vi "小三轮的 FPGA Main Default.vi"() -> ()   [LabVIEW 2017]
doc: "The myRIO v1.1 FPGA Shipping Personality. This personality contains support for:\n- 2 Analog Input Interrupt channel\n- 4 Digital Input Interrupt channel\n- 1 Timer\n- 1 Accelerometer\n- 1 Button\n- 4 LED\n- 10 Analog Input channels with 1 Sample\n- 6 Analog Output channels with 1 Sample\n- 40 Digital I/O channels with 1 Sample\n- 2 I2C channels\n- 4 Encoder channels\n- 6 PWM channels\n- 2 SPI channels"
uses:
  <vilib>/Platform/TimedLoop/XDataNode/timing_clust.ctl
  <vilib>/Platform/TimedLoop/XDataNode/nitl_modes.ctl
  <vilib>/Platform/TimedLoop/XDataNode/wakeup.ctl
  <vilib>/rvi/Emulation/niFpgaGetClockAttributes.vi
  <vilib>/rvi/Emulation/niFpgaSctlEmulationGetInTimedLoop.vi
  <vilib>/rvi/Emulation/niFpgaEmulationReportErrorSimple.vi
  <vilib>/rvi/eio/common/nirviEmuTemplateMethod_errors.vi
  <vilib>/rvi/Emulation/niFpgaCriticalErrorInLSC.vi
  <vilib>/rvi/Emulation/niFpgaProcessEmulError.vi
  <vilib>/rvi/Emulation/niFpgaEmulationIsFPGAContextNoSignature.vi
  <vilib>/rvi/errors/niFpgaSetErrorForExecOnDevCompSimple.vi
  <vilib>/rvi/eio/common/nirviEmuReportErrorAndStop.vi
  <vilib>/rvi/DataTransferAndStorage/Container/Common/niFpgaContainerGetUniqueNameForEmu.vi
  <vilib>/rvi/FIFO/Fifo_Resource/nirvififoEmulationSetSize.vi
  <vilib>/rvi/FIFO/Fifo_Resource/nirviFifoEmulationQueueMgr.vi
  <instcachedir>/0/nirviFifoEmulationQueueMgr_E5CAEC123FF24DC58D834DCA3CDAA9B5.lvgen/nirviFifoEmulationQueueMgr_E5CAEC123FF24DC58D834DCA3CDAA9B5_002.vi
  <vilib>/rvi/FIFO/Fifo_Resource/nirvififoEmulationDetermineInputValidOut.vi
  <vilib>/rvi/FIFO/Fifo_Resource/nirvififoEmulationCreateLock.vi
  <vilib>/rvi/FIFO/Fifo_Resource/nirvififoEmulationObtainLock.vi
  <vilib>/rvi/FIFO/Fifo_Resource/nirvififoEmulationReleaseLock.vi
  <vilib>/rvi/occurrence/nirviWaitOnOccurrenceBase.vi
  <vilib>/rvi/errors/nirviReportUnexpectedCaseInternalError.vi
  <vilib>/rvi/errors/nirviReportUnexpectedCaseInternalError (U32).vi
  <vilib>/Utility/error.llb/Clear Errors.vi
  <vilib>/rvi/DataTransferAndStorage/Container/Common/niFpgaContainerSetEmuInfo.vi
  <vilib>/eio/EIONode/EIONode.xnode
  <vilib>/rvi/DataTransferAndStorage/Container/XNode/niFpgaContainer.xnode
  <vilib>/rvi/FIFO/Fifo_Resource/nirvififoEmulationWrite.vi
  <vilib>/rvi/FIFO/Fifo_Resource/nirvififoEmulationRead.vi
  <vilib>/Platform/TimedLoop/XDataNode/XDataNode.xnode
  <vilib>/rvi/LocalResourceManager/LocalResourceManager.xnode
  <vilib>/Platform/TimedLoop/XDataNode/XDNodeRunTimeDep.lvlib
panel:
  out "timed out? 2":bool
  out "pulse width (uSec) 2":u32
  out "pulse width (uSec)":u32
  out "timed out?":bool
  in  "Reset ENC":bool
  out "ENC2":i32
  out "ENC1":i32
  in  "AO.A_0.VAL":u16
  in  "AO.A_1.VAL":u16
  in  "AO.B_0.VAL":u16
  in  "AO.B_1.VAL":u16
  out "AI.B_3.VAL":u16
  out "AI.B_2.VAL":u16
  out "AI.B_1.VAL":u16
  out "AI.B_0.VAL":u16
  out "AI.A_3.VAL":u16
  out "AI.A_2.VAL":u16
  out "AI.A_1.VAL":u16
  out "AI.A_0.VAL":u16
  out "DIO.B_7:0.IN":u8 format="%08b"
  in  "DIO.B_7:0.DIR":u8 format="%08b"
  in  "DIO.B_7:0.OUT":u8 format="%08b"
  in  "PWM.A_2.CS":u8=1
  in  "PWM.A_2.CNFG":u8=4
  out "PWM.A_2.CNTR":u16
  in  "PWM.A_2.MAX":u16=39999
  in  "PWM.A_2.CMP":u16=20000
  in  "PWM.A_1.CS":u8=1
  in  "PWM.A_1.CNFG":u8=4
  out "PWM.A_1.CNTR":u16
  in  "PWM.A_1.MAX":u16=39999
  in  "PWM.A_1.CMP":u16=20000
  in  "PWM.A_0.CS":u8=1
  in  "PWM.A_0.CNFG":u8=4
  out "PWM.A_0.CNTR":u16
  in  "PWM.A_0.CMP":u16=20000
  in  "PWM.A_0.MAX":u16=39999
  in  "SPI.A.DATO":u16
  out "SPI.A.DATI":u16
  in  "SPI.A.CNFG":u16=112
  in  "SPI.A.CNT":u16=19
  in  "SPI.B.CNT":u16=19
  in  "SPI.B.CNFG":u16=112 format="%0.0f"
  out "SPI.B.DATI":u16
  in  "SPI.B.DATO":u16
  in  "ENC.A.CNFG":u8 format="%08b"
  in  "ENC.B.CNFG":u8 format="%08b"
  out "ENC.A.CNTR":u32
  out "ENC.B.CNTR":u32
  out "ENC.A.STAT":u8 format="%08b"
  out "ENC.B.STAT":u8 format="%08b"
  in  "SPI.A.GO":T1
  out "SPI.A.STAT":u8 format="%08b"
  in  "SPI.B.GO":T1
  out "SPI.B.STAT":u8 format="%08b"
  out "I2C.B.STAT":u8 format="%08b"
  in  "I2C.B.CNTL":u8 format="%08b"
  out "I2C.A.STAT":u8 format="%08b"
  in  "I2C.A.CNTL":u8 format="%08b"
  in  "I2C.B.CNTR":u8=213
  in  "I2C.B.ADDR":u8 format="%08.0f"
  out "I2C.B.DATI":u8
  in  "I2C.B.DATO":u8
  in  "I2C.A.CNTR":u8=213
  in  "I2C.A.ADDR":u8 format="%08b"
  out "I2C.A.DATI":u8
  in  "I2C.A.DATO":u8
  in  "I2C.B.CNFG":u8=1 format="%08b"
  in  "I2C.A.CNFG":u8=1 format="%08b"
  in  "I2C.A.GO":T1
  in  "I2C.B.GO":T1
  out "SYS.AI.RDY":bool
  out "SYS.RDY":bool
  in  "PWM.B_2.CS":u8=1
  in  "PWM.B_2.CNFG":u8=4
  out "PWM.B_2.CNTR":u16
  in  "PWM.B_2.MAX":u16=39999
  in  "PWM.B_2.CMP":u16=20000
  in  "PWM.B_1.CS":u8=1
  in  "PWM.B_1.CNFG":u8=4
  out "PWM.B_1.CNTR":u16
  in  "PWM.B_1.MAX":u16=39999
  in  "PWM.B_1.CMP":u16=20000
  in  "PWM.B_0.CS":u8=1
  in  "PWM.B_0.CNFG":u8=4
  out "PWM.B_0.CNTR":u16
  in  "PWM.B_0.MAX":u16=39999
  in  "PWM.B_0.CMP":u16=20000
  out "DIO.A_7:0.IN":u8 format="%08b"
  in  "DIO.A_7:0.OUT":u8 format="%08b"
  in  "DIO.A_7:0.DIR":u8 format="%08b"
  out "DIO.C_7:0.IN":u8 format="%08b"
  in  "DIO.C_7:0.DIR":u8 format="%08b"
  in  "DIO.C_7:0.OUT":u8 format="%08b"
  out "AI.C_1.VAL":u16
  out "AI.C_0.VAL":u16
  in  "AO.C_0.VAL":u16
  in  "AO.C_1.VAL":u16
  in  "SYS.SELECTB":u8 format="%08b"
  in  "SYS.SELECTC":u8 format="%08b"
  in  "SYS.SELECTA":u8 format="%08b"
  in  "ENC.C_0.CNFG":u8 format="%08b"
  out "ENC.C_0.CNTR":u32
  out "ENC.C_0.STAT":u8 format="%08b"
  in  "ENC.C_1.CNFG":u8 format="%08b"
  out "ENC.C_1.CNTR":u32
  out "ENC.C_1.STAT":u8 format="%08b"
  in  "PWM.C_1.CS":u8=1
  in  "PWM.C_1.CNFG":u8=4
  out "PWM.C_1.CNTR":u16
  in  "PWM.C_1.CMP":u16=20000
  in  "PWM.C_1.MAX":u16=39999
  in  "PWM.C_0.CS":u8=1
  in  "PWM.C_0.CNFG":u8=4
  out "PWM.C_0.CNTR":u16
  in  "PWM.C_0.CMP":u16=20000
  in  "PWM.C_0.MAX":u16=39999
  out "DIO.A_15:8.IN":u8 format="%08b"
  in  "DIO.A_15:8.OUT":u8 format="%08b"
  in  "DIO.A_15:8.DIR":u8 format="%08b"
  out "DIO.B_15:8.IN":u8 format="%08b"
  in  "DIO.B_15:8.DIR":u8 format="%08b"
  in  "DIO.B_15:8.OUT":u8 format="%08b"
  out "AI.AudioIn_R.VAL":u16
  out "AI.AudioIn_L.VAL":u16
  in  "AO.AudioOut_R.VAL":u16
  in  "AO.AudioOut_L.VAL":u16
  in  "AO.SYS.GO":T1
  out "AO.SYS.STAT":bool
  in  "IRQ.AI_A_3:0.CNFG":u8 format="%.0b"
  in  "IRQ.AI_A_0.THRESHOLD":u16
  in  "IRQ.AI_A_1.THRESHOLD":u16
  in  "IRQ.AI_A_0.NO":u8
  in  "IRQ.AI_A_1.NO":u8
  in  "IRQ.DIO_A_7:0.ENA":u8 format="%08b"
  in  "IRQ.DIO_A_7:0.RISE":u8 format="%08b"
  in  "IRQ.DIO_A_7:0.FALL":u8 format="%08b"
  in  "IRQ.DIO_A_0.NO":u8
  in  "IRQ.DIO_A_1.NO":u8
  in  "IRQ.DIO_A_2.NO":u8
  in  "IRQ.DIO_A_3.NO":u8
  in  "IRQ.DIO_A_3.CNT":u32
  in  "IRQ.DIO_A_2.CNT":u32
  in  "IRQ.DIO_A_1.CNT":u32
  in  "IRQ.DIO_A_0.CNT":u32
  in  "IRQ.AI_A_1.HYSTERESIS":u16=17
  in  "IRQ.TIMER.WRITE":u32
  in  "IRQ.TIMER.SETTIME":T1
  out "IRQ.TIMER.READ":u32
  in  "SPI.A.IRQ.NO":u8=15
  in  "SPI.B.IRQ.NO":u8=15
  in  "IRQ.AI_A_0.HYSTERESIS":u16=17
  # "System"
  # "Onboard Devices"
  # "Connector A"
  # "Connector B"
  # "Connector C"
  # "Audio Connector"
  # "Accelerometer"
  # "Analog Input"
  # "Analog Output"
  # "Digital I/O"
  # "PWM"
  # "SPI Master"
  # "Analog Input"
  # "Analog Output"
  # "Digital I/O"
  # "PWM"
  # "SPI Master"
  # "Analog Input"
  # "Analog Output"
  # "Digital I/O"
  # "Counters / PWM"
  # "Analog Input"
  # "Analog Output"
  # "IO Configuration"
  # "IO Configuration"
  # "IO Configuration"
  # "Encoders"
  # "Buttons & LEDs"
  # "Analog Interrupt"
  # "Digital Interrupt"
  # "Encoders"
  # "Encoders"
  # "Button Interrupt"
  # "I2C Master"
  # "I2C Master"
  # "Timer Interrupt"
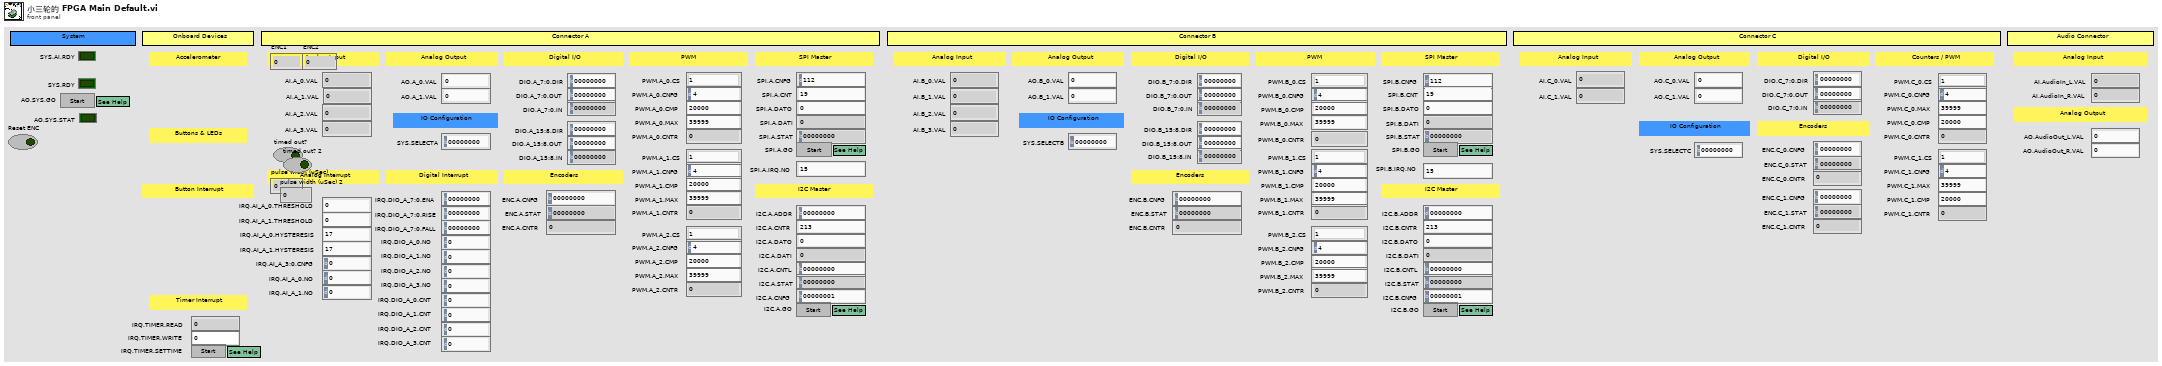
[diagram p1: front panel]
types:
  T1 = typedef "小三轮的 Start Boolean.ctl" = bool
  T2 = typedef "XDNodeRunTimeDep.lvlib/timing_clust.ctl" = cluster{"Expected End [f-1]":u64, "Actual End [f-1]":u64, "Finished Late? [f-1]":bool, "Expected End [i-1]":u64, "Actual End [i-1]":u64, "Finished Late? [i-1]":bool, "Expected Start [i]":u64, "Actual Start [i]":u64, "Expected Start [f]":u64, "Actual Start [f]":u64, "Source Name":string, "Structure Name":string, "Period":i64, "Deadline":i64, "Offset":i64, "Start":i64, "Priority":i32, "Timeout":i32, "Mode":T3, "Wakeup Reason":T4, "Error":errorcluster, "Source Type":string, "Secondary Source Type":string, "Global End Time":u64, "Global Start Time":u64, "Frame Duration":u64, "Iteration Duration":u64, "Assigned CPU":i32, "I/O Scan Engine Mode":u32}
  T3 = typedef "XDNodeRunTimeDep.lvlib/nitl_modes.ctl" = enum32{"No Change", "Process missed periods, maintain original phase", "Discard missed periods, maintain original phase", "Process missed periods, ignore original phase", "Discard missed periods, ignore original phase"}
  T4 = typedef "XDNodeRunTimeDep.lvlib/wakeup.ctl" = enum32{"Normal", "Aborted", "Asynchronous wakeup", "Timing source error", "Timed loop error", "Timeout"}
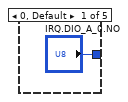
[diagram p6: hidden frame]
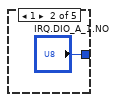
[diagram p7: hidden frame]
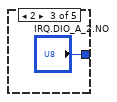
[diagram p8: hidden frame]
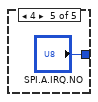
[diagram p9: hidden frame]
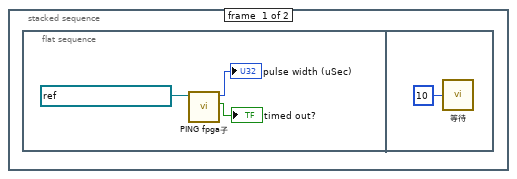
[diagram p10: hidden frame]
diagram:
  # "The Timed Loop does not allow writing the same FIFO outside the Timed Loop. Use another FIFO to push all interrupts from DIO in the Timed Loop to the IRQ Queue."
  # "The Timed Loop does not allow writing the same FIFO outside the Timed Loop. Use another FIFO to push all interrupts from DIO in the Timed Loop to the IRQ Queue."
  # "The analog output nodes take some time before the FPGA write the values to the pins. The GO and STAT registers are used to handshake between the FPGA and host. When the host wants the values to be written, the host sets the GO register to TRUE. If the host reads the STAT register before setting the value of the GO register, it can wait for the value of the STAT register to invert. The value inversion tells the host that the output values have been written."
  # "The analog input nodes take some time before the FPGA can first read the values. This is because it takes time to set up the Analog-to-Digital converter (ADC) and convert the first reading. An iteration of the While Loop will not complete until all the analog input channels have been sampled.\n\nAfter the completion of the first iteration of the While Loop, all indicators have valid values."
  # "Note: On some hardware a \"ghosting effect\" may occur on any unconnected AI channels. For example, if channel AI0 is connected and channels AI1~AI7 are not connected the the value read at AI0 may be seen on indicators AI1~AI7. This is common for hardware that use a multiplexed (MUXed) Analog-to-Digital converter (ADC), because the input analog signal is used to charge a capacitor which does not discharge before the unconnected channel is read.\n\nYou can hide the \"ghosting effect\" by using an mask register. This register is used to decide when the indicator should be updated."
  # "The FPGA timer fires the interrupt request (IRQ) when TIMER.Read counts down to zero. If TIMER.Read is not zero, it counts down to one per microsecond."
  # "The only interface that sends interrupts to the RT side. Timer interrupts, analog input interrupts, digital input interrupts, and SPI interrupt share this interface.\n\nAll interrupts work in sequence. One interrupt waits until the previous interrupt request (IRQ) gets acknowledged on the RT side."
  # "NOTE: The SYS.RDY Boolean MUST exist and must become TRUE at some point. Otherwise, the myRIO VIs will not function correctly."
  # "There is some delay between the time when the FPGA code starts and the time when the analog inputs, accelerometer, and scaling values outputs are valid. If the host wants to ensure that there are valid values in theses registers it should wait for each subsystem to finish its initialization process. \n\nWhen all subsystems have finished initializinig, the SYS.RDY indicator turns true. The host can poll the SYS.RDY indicator to determine the status of the FPGA. Alternatively, the host can poll the individual SYS.xx.RDY indicators to determine the status of the individual subsystems.\n\nThis loop continues indefinitely, essentially making SYS.RDY a read-only register."
  n1 = while {
    stop <- FALSE stop-if-true
    # "Host Synchronization"
    n2 = local read "SYS.AI.RDY"() -> (→"SYS.RDY":bool)
  }
  n3 = while {
    stop <- FALSE stop-if-true
    # "Interrupt to RT"
    n4 = xnode ("FIFO Method Node")("超时"=-1 ("Timeout")) -> ("元素"=w13:u8)  [unwired: 1 in, 2 out]
    n5 = call <vilib>:"niFPGA Interrupt.vi"("Wait Until Cleared (F)"=TRUE, "IRQ Number (0)"=w13) -> ()  [unwired: 1 in]
  }
  n6 = while {
    stop <- FALSE stop-if-true
    # "Timer"
    n7 = local read "IRQ.TIMER.READ"() -> (w18:u32)
    n8 = Select(t="IRQ.TIMER.WRITE", s="IRQ.TIMER.SETTIME", f=w18) -> (s? t:f=w16:u32)
    n9 = case shown="默认" w16 {
      selector: w16 -> [w22 w25]
      tunnel: [w22 w23] -> w15
      frame 0 {
      }
      frame Default {
        n10 = Decrement(x=w25) -> (x-1=w24:u32)
        n11 = case shown="0" w24 {
          selector: w24 -> [w26 w29]
          tunnel: [w26 w29] -> w23
          frame Default {
          }
          frame 0 {
            w28 = u8 0  # Reserved for Timer IRQ
            n12 = xnode ("FIFO Method Node")("元素"=w28, "超时"=-1 ("Timeout")) -> ()  [unwired: 1 in, 2 out]
          }
        }
      }
    }
    "IRQ.TIMER.READ" <- w15
    n13 = call "Loop Timer"("Count(uSec)"=u8 1 ("Count(mSec)")) -> ()  [unwired: 1 out]
  }
  n14 = xnode "通过VI定义FIFO配置"() -> ("FIFO输出"=w2:refnum<k21>)
  n15 = while {
    tunnel: w2 -> [w31]
    i -> [w58]
    stop <- FALSE stop-if-true
    # "Analog Input"
    n16 = xnode "FPGA I/O节点"() -> ("ConnectorA/AI0"=w36:u16, "ConnectorA/AI1"=w35:u16, "ConnectorA/AI2"=→"AI.A_2.VAL":u16, "ConnectorA/AI3"=→"AI.A_3.VAL":u16, "ConnectorB/AI0"=→"AI.B_0.VAL":u16, "ConnectorB/AI1"=→"AI.B_1.VAL":u16, "ConnectorB/AI2"=→"AI.B_2.VAL":u16, "ConnectorB/AI3"=→"AI.B_3.VAL":u16, "ConnectorC/AI0"=w52:i16, "ConnectorC/AI1"=w51:i16, "AudioIn/Left"=w50:i16, "AudioIn/Right"=w49:i16)  [unwired: 12 in, 12 out]
    "AI.A_0.VAL" <- w36
    "AI.A_1.VAL" <- w35
    n17 = Greater Than 0?(x=w58) -> (x > 0?=→"SYS.AI.RDY":bool)
    n18 = Number To Boolean Array(number="IRQ.AI_A_3:0.CNFG") -> (Boolean array=w46:bool[])
    n19 = Index Array(array=w46) -> (element #1=w44:bool, element #2=w43:bool, element #3=w41:bool, element #4=w40:bool)  [unwired: 4 in]
    n20 = To Unsigned Word Integer(number=w52) -> (unsigned 16bit integer=→"AI.C_0.VAL":u16)
    n21 = To Unsigned Word Integer(number=w51) -> (unsigned 16bit integer=→"AI.C_1.VAL":u16)
    n22 = To Unsigned Word Integer(number=w50) -> (unsigned 16bit integer=→"AI.AudioIn_L.VAL":u16)
    n23 = To Unsigned Word Integer(number=w49) -> (unsigned 16bit integer=→"AI.AudioIn_R.VAL":u16)
    n24 = call "小三轮的 Check AI IRQ.vi"("Hysteresis"="IRQ.AI_A_1.HYSTERESIS", "FIFO In"=w31, "IRQ Number"="IRQ.AI_A_1.NO", "Threshold"="IRQ.AI_A_1.THRESHOLD", "Analog Value"=w35, "Rising Edge?"=w40, "Enable Interrupt?"=w41) -> ()  [unwired: 5 in]
    n25 = call "小三轮的 Check AI IRQ.vi"("Hysteresis"="IRQ.AI_A_0.HYSTERESIS", "FIFO In"=w31, "IRQ Number"="IRQ.AI_A_0.NO", "Threshold"="IRQ.AI_A_0.THRESHOLD", "Analog Value"=w36, "Rising Edge?"=w43, "Enable Interrupt?"=w44) -> ()  [unwired: 5 in]
  }
  n26 = while {
    stop <- FALSE stop-if-true
    # "Analog Output"
    n27 = feedback #1(FALSE) -> (w64:bool)
    n28 = case shown="真" "AO.SYS.GO" {
      tunnel: "AO.C_0.VAL" -> [_ w86]
      tunnel: "AO.C_1.VAL" -> [_ w85]
      tunnel: "AO.A_0.VAL" -> [_ w90]
      tunnel: "AO.A_1.VAL" -> [_ w89]
      tunnel: "AO.B_0.VAL" -> [_ w88]
      tunnel: "AO.B_1.VAL" -> [_ w87]
      tunnel: "AO.AudioOut_L.VAL" -> [_ w82]
      tunnel: "AO.AudioOut_R.VAL" -> [_ w81]
      tunnel: w64 -> [w75 w78]
      tunnel: [w75 w76] -> w62
      frame False {
      }
      frame True {
        n29 = To Word Integer(number=w86) -> (16bit integer=w84:i16)
        n30 = To Word Integer(number=w85) -> (16bit integer=w83:i16)
        n31 = To Word Integer(number=w82) -> (16bit integer=w80:i16)
        n32 = To Word Integer(number=w81) -> (16bit integer=w79:i16)
        n33 = flat-sequence {
          tunnel: w90 -> [w99]
          tunnel: w89 -> [w98]
          tunnel: w88 -> [w97]
          tunnel: w87 -> [w96]
          tunnel: w84 -> [w95]
          tunnel: w83 -> [w94]
          tunnel: w80 -> [w93]
          tunnel: w79 -> [w92]
          tunnel: w78 -> [w91]
          tunnel: [w91] -> w77
          tunnel: w77 -> [w101]
          tunnel: [w100] -> w76
          frame #0 {
            n34 = xnode "FPGA I/O节点"("ConnectorA/AO0"=w99, "ConnectorA/AO1"=w98, "ConnectorB/AO0"=w97, "ConnectorB/AO1"=w96, "ConnectorC/AO0"=w95, "ConnectorC/AO1"=w94, "AudioOut/Left"=w93, "AudioOut/Right"=w92) -> ()  [unwired: 8 in, 8 out]
          }
          frame #1 {
            n35 = Not(x=w101) -> (.not. x?=w100:bool)
          }
        }
      }
    }
    "AO.SYS.STAT" <- w62
    n36 = feedback-in #1(w62) -> ()
  }
  n37 = while {
    stop <- FALSE stop-if-true
    # "PING)))"
    n38 = stacked-sequence {
      frame #0 {
        n39 = flat-sequence {
          frame #0 {
            n40 = call "PING fpga子.vi"("引用句柄输入"=refnum<k21> "ConnectorB/DIO0") -> ("timed out?"=→"timed out?":bool, "pulse width (uSec)"=→"pulse width (uSec)":u32)  [unwired: 9 in]
          }
          frame #1 {
            n41 = call "等待"("Count(uSec)"=u32 10) -> ()  [unwired: 1 out]
          }
        }
      }
      frame #1 {
        n42 = flat-sequence {
          frame #0 {
            n43 = call "PING fpga子.vi"("引用句柄输入"=refnum<k21> "ConnectorB/DIO1") -> ("timed out?"=→"timed out? 2":bool, "pulse width (uSec)"=→"pulse width (uSec) 2":u32)  [unwired: 9 in]
          }
          frame #1 {
            n44 = call "等待2"("Count(uSec)"=u32 10) -> ()  [unwired: 1 out]
          }
        }
      }
    }
  }
  n45 = while {
    stop <- FALSE stop-if-true
    # "Encode"
    n46 = xnode "FPGA I/O节点"() -> ("ConnectorA/DIO0"=w118:bool, "ConnectorA/DIO1"=w117:bool, "ConnectorA/DIO2"=w116:bool, "ConnectorA/DIO3"=w115:bool)  [unwired: 4 in, 4 out]
    n47 = call "FPGA Encode.vi"("Reset ENC1"="Reset ENC", "B"=w117, "A"=w118) -> ("ENC"=→"ENC1":i32)  [unwired: 8 in]
    n48 = call "FPGA Encode.vi"("Reset ENC1"="Reset ENC", "B"=w115, "A"=w116) -> ("ENC"=→"ENC2":i32)  [unwired: 8 in]
  }
  n49 = node-c288() -> (w6:T2)  [unwired: 1 in]
  n50 = xnode "通过VI定义FIFO配置"() -> ()  [unwired: 1 out]
  n51 = while {
    stop <- FALSE stop-if-true
    # "Connector A SCTL Interrupt Buffer"
    n52 = feedback #2(u8 0 ("Element")) -> (w121:u8)
    n53 = feedback #3(FALSE ("Timed Out?")) -> (w125:bool)
    n54 = case shown="假" w125 {
      tunnel: [w127 w129] -> w122
      tunnel: w121 -> [_ w129]
      frame False {
        n55 = xnode ("FIFO Method Node")("超时"=-1 ("Timeout")) -> ("元素"=w127:u8)  [unwired: 1 in, 2 out]
      }
      frame True {
      }
    }
    n56 = feedback-in #2(w122) -> ()
    n57 = xnode ("FIFO Method Node")("元素"=w122, "超时"=0 ("Timeout")) -> ("超时？"=w123:bool)  [unwired: 1 in, 1 out]
    n58 = feedback-in #3(w123) -> ()
  }
  n59 = timed-loop {
    timing: w6 -> [_]
    timing-out: [_] -> w5
    stop <- _ stop-if-true
    w153 = fxp<+,4,4> 0.0 ("IN 3:0")
    w130 = u16 5 ("Debounce Ticks")
    w131 = u8 0
    # "Trigger the interrupt at next \ntick if timeout"
    # "DIO / Encoder"
    # "DIO / I2C Master"
    # "DIO / PWM"
    # "DIO"
    # "DIO"
    # "DIO/ SPI Master"
    # "Connector A DIO"
    n60 = call "小三轮的 Split HDC Bank1 DIO.vi"("IN 7:0"="DIO.A_7:0.OUT") -> ("OUT 4"=w185:bool, "OUT 7:5"=w259:fxp<+,3,3>)  [unwired: 1 out]
    n61 = call "小三轮的 Split HDC Bank1 DIO.vi"("IN 7:0"="DIO.A_7:0.DIR") -> ("OUT 4"=w260:bool, "OUT 7:5"=w258:fxp<+,3,3>)  [unwired: 1 out]
    n62 = call "小三轮的 Split HDC Function Select.vi"("IN 7:0"="SYS.SELECTA") -> ("OUT 1:0"=w205:fxp<+,2,2>, "OUT 7"=w200:bool, "OUT 2"=w204:bool, "OUT 3"=w203:bool, "OUT 4"=w202:bool, "OUT 5"=w201:bool)
    n63 = call "小三轮的 DIO 1-bit.vi"("DIR"=w260, "OUT"=w185, "DIO Refnum"=refnum<k21> "ConnectorA/DIO4") -> ("IN"=w152:bool)  [unwired: 8 in]
    n64 = call "小三轮的 DIO_SPI.vi"("DIO.2:0.OUT"=w259, "DIO.2:0.DIR"=w258, "SPI.CNT"="SPI.A.CNT", "SPI.CNFG"="SPI.A.CNFG", "SPI.DATO"="SPI.A.DATO", "SPI.GO"="SPI.A.GO", "DIO.2/SPI.MOSI Refnum"=refnum<k21> "ConnectorA/DIO7" ("DIO.2/SPI.SCLK"), "SELECT.1:0"=w205, "DIO.1/SPI.MISO Refnum"=refnum<k21> "ConnectorA/DIO6" ("DIO.1/SPI.MOSI"), "DIO.0/SPI.SCLK Refnum"=refnum<k21> "ConnectorA/DIO5" ("DIO.0/SPI.MISO")) -> ("DIO.2:0.IN"=w238:fxp<+,3,3>, "SPI.DATI"=→"SPI.A.DATI":u16, "SPI.STAT"=w138:u8)  [unwired: 7 in]
    "SPI.A.STAT" <- w138
    n65 = Number To Boolean Array(number=w138) -> (Boolean array=w140:bool[])
    n66 = Index Array(array=w140) -> (element=w139:bool)  [unwired: 1 in]
    n67 = call "小三轮的 Falling Edge Trigger.vi"("Signal"=w139) -> ("Trigger?"=w137:bool)
    n68 = call "小三轮的 Join HDC Bank1 DIO.vi"("IN 7:5"=w238, "IN 4"=w152, "IN 3:0"=w153) -> ("OUT 7:0"=→"DIO.A_7:0.IN":u8)
    n69 = Number To Boolean Array(number=w153) -> (Boolean array=w178:bool[])
    n70 = Number To Boolean Array(number="IRQ.DIO_A_7:0.ENA") -> (Boolean array=w184:bool[])
    n71 = Number To Boolean Array(number="IRQ.DIO_A_7:0.RISE") -> (Boolean array=w183:bool[])
    n72 = Number To Boolean Array(number="IRQ.DIO_A_7:0.FALL") -> (Boolean array=w182:bool[])
    n73 = call "小三轮的 Split HDC Bank2 DIO.vi"("IN 7:0"="DIO.A_15:8.OUT") -> ("OUT 5"=w187:bool, "OUT 7:6"=w209:fxp<+,2,2>, "OUT 4:3"=w189:fxp<+,2,2>, "OUT 2"=w191:bool, "OUT 0"=w195:bool, "OUT 1"=w194:bool)  [unwired: 2 in]
    n74 = call "小三轮的 Split HDC Bank2 DIO.vi"("IN 7:0"="DIO.A_15:8.DIR") -> ("OUT 5"=w186:bool, "OUT 7:6"=w208:fxp<+,2,2>, "OUT 4:3"=w188:fxp<+,2,2>, "OUT 2"=w190:bool, "OUT 0"=w193:bool, "OUT 1"=w192:bool)  [unwired: 2 in]
    n75 = Index Array(array=w178) -> (element #1=w159:bool, element #2=w174:bool, element #3=w173:bool, element #4=w172:bool)  [unwired: 4 in]
    n76 = Index Array(array=w184) -> (element #1=w177:bool, element #2=w171:bool, element #3=w170:bool, element #4=w169:bool)  [unwired: 4 in]
    n77 = Index Array(array=w183) -> (element #1=w176:bool, element #2=w168:bool, element #3=w167:bool, element #4=w166:bool)  [unwired: 4 in]
    n78 = Index Array(array=w182) -> (element #1=w175:bool, element #2=w165:bool, element #3=w164:bool, element #4=w163:bool)  [unwired: 4 in]
    n79 = call "小三轮的 Check DI IRQ.vi"("Debounce Ticks"=w130, "Count"="IRQ.DIO_A_0.CNT", "On Falling Edge?"=w175, "On Rising Edge?"=w176, "Enable Interrupt?"=w177, "Digital In"=w159) -> ("Trigger?"=w150:bool)  [unwired: 5 in]
    n80 = call "小三轮的 Check DI IRQ.vi"("Debounce Ticks"=w130, "Count"="IRQ.DIO_A_1.CNT", "On Falling Edge?"=w165, "On Rising Edge?"=w168, "Enable Interrupt?"=w171, "Digital In"=w174) -> ("Trigger?"=w149:bool)  [unwired: 5 in]
    n81 = call "小三轮的 Check DI IRQ.vi"("Debounce Ticks"=w130, "Count"="IRQ.DIO_A_2.CNT", "On Falling Edge?"=w164, "On Rising Edge?"=w167, "Enable Interrupt?"=w170, "Digital In"=w173) -> ("Trigger?"=w148:bool)  [unwired: 5 in]
    n82 = call "小三轮的 DIO_PWM.vi"("DIO.OUT"=w195, "DIO.DIR"=w193, "PWM.CS"="PWM.A_0.CS", "PWM.CNFG"="PWM.A_0.CNFG", "PWM.CMP"="PWM.A_0.CMP", "PWM.MAX"="PWM.A_0.MAX", "DIO/PWM"=refnum<k21> "ConnectorA/DIO8", "SELECT"=w204) -> ("DIO.IN"=w199:bool, "PWM.CNTR"=→"PWM.A_0.CNTR":u16)  [unwired: 10 in]
    n83 = call "小三轮的 DIO_PWM.vi"("DIO.OUT"=w194, "DIO.DIR"=w192, "PWM.CS"="PWM.A_1.CS", "PWM.CNFG"="PWM.A_1.CNFG", "PWM.CMP"="PWM.A_1.CMP", "PWM.MAX"="PWM.A_1.MAX", "DIO/PWM"=refnum<k21> "ConnectorA/DIO9", "SELECT"=w203) -> ("DIO.IN"=w198:bool, "PWM.CNTR"=→"PWM.A_1.CNTR":u16)  [unwired: 10 in]
    n84 = call "小三轮的 DIO_PWM.vi"("DIO.OUT"=w191, "DIO.DIR"=w190, "PWM.CS"="PWM.A_2.CS", "PWM.CNFG"="PWM.A_2.CNFG", "PWM.CMP"="PWM.A_2.CMP", "PWM.MAX"="PWM.A_2.MAX", "DIO/PWM"=refnum<k21> "ConnectorA/DIO10", "SELECT"=w202) -> ("DIO.IN"=w197:bool, "PWM.CNTR"=→"PWM.A_2.CNTR":u16)  [unwired: 10 in]
    n85 = call "小三轮的 Check DI IRQ.vi"("Debounce Ticks"=w130, "Count"="IRQ.DIO_A_3.CNT", "On Falling Edge?"=w163, "On Rising Edge?"=w166, "Enable Interrupt?"=w169, "Digital In"=w172) -> ("Trigger?"=w147:bool)  [unwired: 5 in]
    n86 = feedback #4(w131) -> (w133:u8)
    n87 = Less?(x=w133, y=4 ("x")) -> (x < y?=w135:bool)
    n88 = Increment(x=w133) -> (x+1=w134:u8)
    n89 = Select(t=w134, s=w135, f=w131) -> (s? t:f=w132:u8)
    n90 = feedback-in #4(w132) -> ()
    n91 = case shown="3" w133 {
      tunnel: ["IRQ.DIO_A_0.NO" "IRQ.DIO_A_1.NO" "IRQ.DIO_A_2.NO" "IRQ.DIO_A_3.NO" "SPI.A.IRQ.NO"] -> w162
      frame 0, Default {
      }
      frame 1 {
      }
      frame 2 {
      }
      frame 3 {
      }
      frame 4 {
      }
    }
    n92 = Build Array(w150, w149, w148, w147, w137) -> (w145:bool[])
    n93 = call "小三轮的 DIO_Encoder.vi"("DIO.1:0.OUT"=w189, "DIO.1:0.DIR"=w188, "QE.CNFG"="ENC.A.CNFG", "DIO.1/QE.B"=refnum<k21> "ConnectorA/DIO12", "SELECT"=w201, "DIO.0/QE.A"=refnum<k21> "ConnectorA/DIO11") -> ("DIO.1:0.IN"=w196:fxp<+,2,2>, "QE.CNTR"=→"ENC.A.CNTR":u32, "QE.STAT"=→"ENC.A.STAT":u8)  [unwired: 11 in]
    n94 = call "小三轮的 DIO 1-bit.vi"("DIR"=w186, "OUT"=w187, "DIO Refnum"=refnum<k21> "ConnectorA/DIO13") -> ("IN"=w151:bool)  [unwired: 8 in]
    n95 = call "小三轮的 DIO_I2C.vi"("DIO.1:0.OUT"=w209, "DIO.1:0.DIR"=w208, "I2C.CNFG"="I2C.A.CNFG", "I2C.CNTL"="I2C.A.CNTL", "I2C.ADDR"="I2C.A.ADDR", "I2C.DATO"="I2C.A.DATO", "DIO.1/I2C.SDA"=refnum<k21> "ConnectorA/DIO15" ("DIO.1/I2C.SCL"), "I2C.CNTR"="I2C.A.CNTR", "DIO.0/I2C.SCL"=refnum<k21> "ConnectorA/DIO14" ("DIO.0/I2C.SDA"), "Execute?"="I2C.A.GO", "SELECT"=w200) -> ("DIO.1:0.IN"=w207:fxp<+,2,2>, "I2C.DATI"=→"I2C.A.DATI":u8, "I2C.STAT"=→"I2C.A.STAT":u8)  [unwired: 6 in]
    n96 = feedback #5(bool[] [FALSE, FALSE, FALSE, FALSE, FALSE] ("initialized array")) -> (w141:bool[])
    n97 = Or(x=w145, y=w141) -> (x .or. y?=w146:bool[])
    n98 = Index Array(array=w146, index=w133) -> (element=w144:bool)
    n99 = case shown="真" w144 {
      selector: w144 -> [w261 _]
      tunnel: [w261 w262] -> w143
      tunnel: w162 -> [_ w263]
      frame False {
      }
      frame True {
        n100 = xnode ("FIFO Method Node")("元素"=w263, "超时"=0 ("Timeout")) -> ("超时？"=w262:bool)  [unwired: 1 in, 1 out]
      }
    }
    n101 = Replace Array Subset(array=w146, new element=w143, index=w133) -> (w142:bool[])
    n102 = feedback-in #5(w142) -> ()
    n103 = call "小三轮的 Join HDC Bank2 DIO.vi"("IN 7:6"=w207, "IN 5"=w151, "IN 4:3"=w196, "IN 0"=w199, "IN 2"=w197, "IN 1"=w198) -> ("OUT 7:0"=→"DIO.A_15:8.IN":u8)  [unwired: 4 in]
  }
  n104 = node-c288(w5) -> ()
  n105 = xnode "通过VI定义FIFO配置"() -> ("FIFO输出"=w1:refnum<k21>)
  n106 = node-c288() -> (w4:T2)  [unwired: 1 in]
  n107 = timed-loop {
    timing: w4 -> [_]
    timing-out: [_] -> w3
    tunnel: w1 -> [w273]
    stop <- _ stop-if-true
    # "DIO / Encoder"
    # "DIO / I2C Master"
    # "DIO / PWM"
    # "DIO"
    # "DIO"
    # "DIO/ SPI Master"
    # "Connector B DIO"
    n108 = call "小三轮的 Split HDC Bank1 DIO.vi"("IN 7:0"="DIO.B_7:0.OUT") -> ("OUT 4"=w355:bool, "OUT 7:5"=w353:fxp<+,3,3>)  [unwired: 1 out]
    n109 = call "小三轮的 Split HDC Bank1 DIO.vi"("IN 7:0"="DIO.B_7:0.DIR") -> ("OUT 4"=w354:bool, "OUT 7:5"=w352:fxp<+,3,3>)  [unwired: 1 out]
    n110 = call "小三轮的 Split HDC Function Select.vi"("IN 7:0"="SYS.SELECTB") -> ("OUT 1:0"=w334:fxp<+,2,2>, "OUT 7"=w329:bool, "OUT 2"=w333:bool, "OUT 3"=w332:bool, "OUT 4"=w331:bool, "OUT 5"=w330:bool)
    n111 = call "小三轮的 DIO 1-bit.vi"("DIR"=w354, "OUT"=w355, "DIO Refnum"=refnum<k21> "ConnectorB/DIO4") -> ("IN"=w339:bool)  [unwired: 8 in]
    n112 = call "小三轮的 DIO_SPI.vi"("DIO.2:0.OUT"=w353, "DIO.2:0.DIR"=w352, "SPI.CNT"="SPI.B.CNT", "SPI.CNFG"="SPI.B.CNFG", "SPI.DATO"="SPI.B.DATO", "SPI.GO"="SPI.B.GO", "DIO.2/SPI.MOSI Refnum"=refnum<k21> "ConnectorB/DIO7" ("DIO.2/SPI.SCLK"), "SELECT.1:0"=w334, "DIO.1/SPI.MISO Refnum"=refnum<k21> "ConnectorB/DIO6" ("DIO.1/SPI.MOSI"), "DIO.0/SPI.SCLK Refnum"=refnum<k21> "ConnectorB/DIO5" ("DIO.0/SPI.MISO")) -> ("DIO.2:0.IN"=w338:fxp<+,3,3>, "SPI.DATI"=→"SPI.B.DATI":u16, "SPI.STAT"=w274:u8)  [unwired: 7 in]
    "SPI.B.STAT" <- w274
    n113 = call "小三轮的 SPI IRQ.vi"("SPI.A.IRQ.NO"="SPI.B.IRQ.NO", "SPI.STAT"=w274, "FIFO In"=w273) -> ()  [unwired: 9 in]
    n114 = call "小三轮的 Join HDC Bank1 DIO.vi"("IN 7:5"=w338, "IN 4"=w339, "IN 3:0"=fxp<+,4,4> 0.0) -> ("OUT 7:0"=→"DIO.B_7:0.IN":u8)
    n115 = call "小三轮的 Split HDC Bank2 DIO.vi"("IN 7:0"="DIO.B_15:8.OUT") -> ("OUT 5"=w286:bool, "OUT 7:6"=w337:fxp<+,2,2>, "OUT 4:3"=w287:fxp<+,2,2>, "OUT 2"=w288:bool, "OUT 0"=w290:bool, "OUT 1"=w289:bool)  [unwired: 2 in]
    n116 = call "小三轮的 Split HDC Bank2 DIO.vi"("IN 7:0"="DIO.B_15:8.DIR") -> ("OUT 5"=w281:bool, "OUT 7:6"=w336:fxp<+,2,2>, "OUT 4:3"=w282:fxp<+,2,2>, "OUT 2"=w283:bool, "OUT 0"=w285:bool, "OUT 1"=w284:bool)  [unwired: 2 in]
    n117 = call "小三轮的 DIO_PWM.vi"("DIO.OUT"=w290, "DIO.DIR"=w285, "PWM.CS"="PWM.B_0.CS", "PWM.CNFG"="PWM.B_0.CNFG", "PWM.CMP"="PWM.B_0.CMP", "PWM.MAX"="PWM.B_0.MAX", "DIO/PWM"=refnum<k21> "ConnectorB/DIO8", "SELECT"=w333) -> ("DIO.IN"=w280:bool, "PWM.CNTR"=→"PWM.B_0.CNTR":u16)  [unwired: 10 in]
    n118 = call "小三轮的 DIO_PWM.vi"("DIO.OUT"=w289, "DIO.DIR"=w284, "PWM.CS"="PWM.B_1.CS", "PWM.CNFG"="PWM.B_1.CNFG", "PWM.CMP"="PWM.B_1.CMP", "PWM.MAX"="PWM.B_1.MAX", "DIO/PWM"=refnum<k21> "ConnectorB/DIO9", "SELECT"=w332) -> ("DIO.IN"=w279:bool, "PWM.CNTR"=→"PWM.B_1.CNTR":u16)  [unwired: 10 in]
    n119 = call "小三轮的 DIO_PWM.vi"("DIO.OUT"=w288, "DIO.DIR"=w283, "PWM.CS"="PWM.B_2.CS", "PWM.CNFG"="PWM.B_2.CNFG", "PWM.CMP"="PWM.B_2.CMP", "PWM.MAX"="PWM.B_2.MAX", "DIO/PWM"=refnum<k21> "ConnectorB/DIO10", "SELECT"=w331) -> ("DIO.IN"=w278:bool, "PWM.CNTR"=→"PWM.B_2.CNTR":u16)  [unwired: 10 in]
    n120 = call "小三轮的 DIO_Encoder.vi"("DIO.1:0.OUT"=w287, "DIO.1:0.DIR"=w282, "QE.CNFG"="ENC.B.CNFG", "DIO.1/QE.B"=refnum<k21> "ConnectorB/DIO12", "SELECT"=w330, "DIO.0/QE.A"=refnum<k21> "ConnectorB/DIO11") -> ("DIO.1:0.IN"=w277:fxp<+,2,2>, "QE.CNTR"=→"ENC.B.CNTR":u32, "QE.STAT"=→"ENC.B.STAT":u8)  [unwired: 11 in]
    n121 = call "小三轮的 DIO 1-bit.vi"("DIR"=w281, "OUT"=w286, "DIO Refnum"=refnum<k21> "ConnectorB/DIO13") -> ("IN"=w276:bool)  [unwired: 8 in]
    n122 = call "小三轮的 DIO_I2C.vi"("DIO.1:0.OUT"=w337, "DIO.1:0.DIR"=w336, "I2C.CNFG"="I2C.B.CNFG", "I2C.CNTL"="I2C.B.CNTL", "I2C.ADDR"="I2C.B.ADDR", "I2C.DATO"="I2C.B.DATO", "DIO.1/I2C.SDA"=refnum<k21> "ConnectorB/DIO15" ("DIO.1/I2C.SCL"), "I2C.CNTR"="I2C.B.CNTR", "DIO.0/I2C.SCL"=refnum<k21> "ConnectorB/DIO14" ("DIO.0/I2C.SDA"), "Execute?"="I2C.B.GO", "SELECT"=w329) -> ("DIO.1:0.IN"=w335:fxp<+,2,2>, "I2C.DATI"=→"I2C.B.DATI":u8, "I2C.STAT"=→"I2C.B.STAT":u8)  [unwired: 6 in]
    n123 = call "小三轮的 Join HDC Bank2 DIO.vi"("IN 7:6"=w335, "IN 5"=w276, "IN 4:3"=w277, "IN 0"=w280, "IN 2"=w278, "IN 1"=w279) -> ("OUT 7:0"=→"DIO.B_15:8.IN":u8)  [unwired: 4 in]
  }
  n124 = while {
    stop <- FALSE stop-if-true
    # "Connector B SCTL Interrupt Buffer"
    n125 = feedback #6(u8 0 ("Element")) -> (w360:u8)
    n126 = feedback #7(FALSE ("Timed Out?")) -> (w364:bool)
    n127 = case shown="假" w364 {
      tunnel: [w366 w368] -> w361
      tunnel: w360 -> [_ w368]
      frame False {
        n128 = xnode ("FIFO Method Node")("超时"=-1 ("Timeout")) -> ("元素"=w366:u8)  [unwired: 1 in, 2 out]
      }
      frame True {
      }
    }
    n129 = feedback-in #6(w361) -> ()
    n130 = xnode ("FIFO Method Node")("元素"=w361, "超时"=0 ("Timeout")) -> ("超时？"=w362:bool)  [unwired: 1 in, 1 out]
    n131 = feedback-in #7(w362) -> ()
  }
  n132 = node-c288(w3) -> ()
  n133 = node-c288() -> (w8:T2)  [unwired: 1 in]
  n134 = timed-loop {
    timing: w8 -> [_]
    timing-out: [_] -> w7
    stop <- _ stop-if-true
    # "Connector C  DIO"
    n135 = call "小三轮的 Split myDAQ DIO.vi"("IN 7:0"="DIO.C_7:0.OUT") -> ("OUT 2, OUT0"=w387:fxp<+,2,2>, "OUT 1"=w386:bool, "OUT 3"=w385:bool, "OUT 7"=w382:bool, "OUT 6, OUT 4"=w384:fxp<+,2,2>, "OUT 5"=w383:bool)  [unwired: 4 in]
    n136 = call "小三轮的 Split myDAQ DIO.vi"("IN 7:0"="DIO.C_7:0.DIR") -> ("OUT 2, OUT0"=w381:fxp<+,2,2>, "OUT 1"=w380:bool, "OUT 3"=w379:bool, "OUT 7"=w376:bool, "OUT 6, OUT 4"=w378:fxp<+,2,2>, "OUT 5"=w377:bool)  [unwired: 4 in]
    n137 = call "小三轮的 Split myDAQ Function Select.vi"("IN 7:0"="SYS.SELECTC") -> ("OUT 0"=w393:bool, "OUT 1"=w392:bool, "OUT 2"=w391:bool, "OUT 3"=w390:bool)  [unwired: 2 in]
    n138 = call "小三轮的 DIO_Encoder.vi"("DIO.1:0.OUT"=w387, "DIO.1:0.DIR"=w381, "QE.CNFG"="ENC.C_0.CNFG", "DIO.1/QE.B"=refnum<k21> "ConnectorC/DIO2", "SELECT"=w393, "DIO.0/QE.A"=refnum<k21> "ConnectorC/DIO0") -> ("DIO.1:0.IN"=w374:fxp<+,2,2>, "QE.CNTR"=→"ENC.C_0.CNTR":u32, "QE.STAT"=→"ENC.C_0.STAT":u8)  [unwired: 11 in]
    n139 = call "小三轮的 DIO 1-bit.vi"("DIR"=w380, "OUT"=w386, "DIO Refnum"=refnum<k21> "ConnectorC/DIO1") -> ("IN"=w373:bool)  [unwired: 8 in]
    n140 = call "小三轮的 DIO_PWM.vi"("DIO.OUT"=w385, "DIO.DIR"=w379, "PWM.CS"="PWM.C_0.CS", "PWM.CNFG"="PWM.C_0.CNFG", "PWM.CMP"="PWM.C_0.CMP", "PWM.MAX"="PWM.C_0.MAX", "DIO/PWM"=refnum<k21> "ConnectorC/DIO3", "SELECT"=w392) -> ("DIO.IN"=w372:bool, "PWM.CNTR"=→"PWM.C_0.CNTR":u16)  [unwired: 10 in]
    n141 = call "小三轮的 DIO_Encoder.vi"("DIO.1:0.OUT"=w384, "DIO.1:0.DIR"=w378, "QE.CNFG"="ENC.C_1.CNFG", "DIO.1/QE.B"=refnum<k21> "ConnectorC/DIO6", "SELECT"=w391, "DIO.0/QE.A"=refnum<k21> "ConnectorC/DIO4") -> ("DIO.1:0.IN"=w371:fxp<+,2,2>, "QE.CNTR"=→"ENC.C_1.CNTR":u32, "QE.STAT"=→"ENC.C_1.STAT":u8)  [unwired: 11 in]
    n142 = call "小三轮的 DIO 1-bit.vi"("DIR"=w377, "OUT"=w383, "DIO Refnum"=refnum<k21> "ConnectorC/DIO5") -> ("IN"=w370:bool)  [unwired: 8 in]
    n143 = call "小三轮的 DIO_PWM.vi"("DIO.OUT"=w382, "DIO.DIR"=w376, "PWM.CS"="PWM.C_1.CS", "PWM.CNFG"="PWM.C_1.CNFG", "PWM.CMP"="PWM.C_1.CMP", "PWM.MAX"="PWM.C_1.MAX", "DIO/PWM"=refnum<k21> "ConnectorC/DIO7", "SELECT"=w390) -> ("DIO.IN"=w369:bool, "PWM.CNTR"=→"PWM.C_1.CNTR":u16)  [unwired: 10 in]
    n144 = call "小三轮的 Join myDAQ DIO.vi"("IN 7"=w369, "IN 5"=w370, "IN 6, IN 4"=w371, "IN 2, IN 0"=w374, "IN 3"=w372, "IN 1"=w373) -> ("IN 7:0"=→"DIO.C_7:0.IN":u8)  [unwired: 4 in]
  }
  n145 = node-c288(w7) -> ()
